vi "Server2.vi"   [LabVIEW 2013]
uses:
  <vilib>/NXT/Block Support/NXT_MessageMailbox.ctl
  <vilib>/NXT/Dual Mode Library/Display/drawText.vi
types:
  T1 = typedef "LVHSConnector.ctl" = refnum<class "BrickReference.lvclass">
  T2 = typedef "NXT_MessageMailbox.ctl" = u8
  T3 = typedef "NXT_InputPort.ctl" = u32
  T4 = typedef "MotorOutput.ctl" = u8
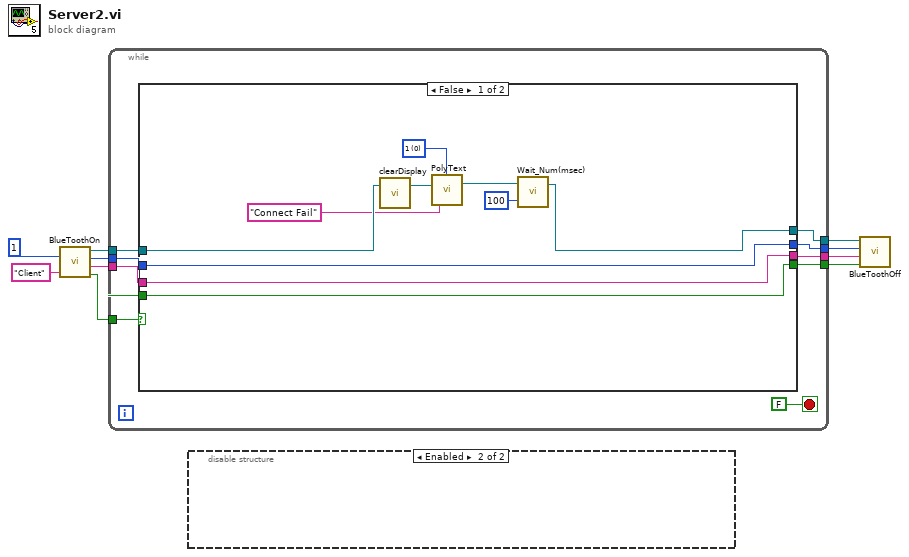
[diagram p0: block diagram]
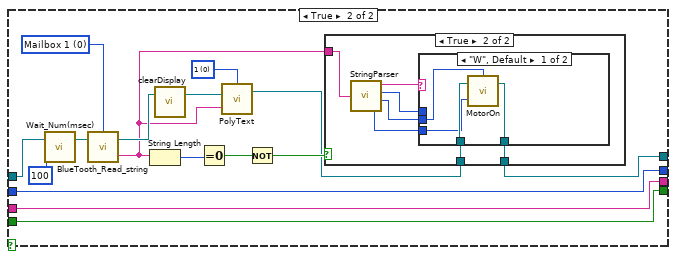
[diagram p2: hidden frame]
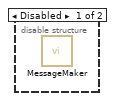
[diagram p5: hidden frame]
diagram:
  n1 = call "BlueToothOn.vi"("Connection"=u8 1, "Partner Name"="Client") -> ("NXT/EV3 2"=w2:T1, "Connection"=w4:u8, "Partner Name"=w7:string, "Success"=w9:bool)  [unwired: 1 in]
  n2 = while {
    tunnel: [w19] -> w10
    tunnel: w9 -> [w18]
    tunnel: w7 -> [w17]
    tunnel: [w16] -> w6
    tunnel: w4 -> [w15]
    tunnel: [w14] -> w3
    tunnel: w2 -> [w13]
    tunnel: [w12] -> w1
    stop <- FALSE stop-if-true
    n3 = case shown="False" w18 {
      tunnel: [w27 w45] -> w19
      tunnel: w18 -> [w27 w45]
      tunnel: w17 -> [w28 w44]
      tunnel: [w28 w44] -> w16
      tunnel: w15 -> [w29 w43]
      tunnel: [w20 w38] -> w14
      tunnel: w13 -> [w24 w37]
      tunnel: [w29 w43] -> w12
      frame False {
        w26 = i16 0 items=["1", "2", "3", "4", "5", "6", "7", "8", "9", "10", "11", "12"] ("Line")
        n4 = call <vilib>:"clearDisplay.vi"("NXT/EV3"=w24) -> ("NXT/EV3"=w25:T1)  [unwired: 3 in]
        n5 = call-poly <vilib>:"PolyText.vi"("Text"="Connect Fail", "NXT/EV3"=w25, "Line"=w26) -> ("NXT/EV3"=w21:T1)  [unwired: 1 in]
        n6 = call <vilib>:"Wait_Num(msec).vi"("Time (100 msec)"=u32 100, "NXT/EV3"=w21) -> ("NXT/EV3"=w20:T1)  [unwired: 2 in]
      }
      frame True {
        w32 = i16 0 items=["1", "2", "3", "4", "5", "6", "7", "8", "9", "10", "11", "12"] ("Line")
        w41 = T2 0 items=["Mailbox 1", "Mailbox 2", "Mailbox 3", "Mailbox 4", "Mailbox 5", "Mailbox 6", "Mailbox 7", "Mailbox 8", "Mailbox 9", "Mailbox 10"] ("Mailbox")
        n7 = call <vilib>:"Wait_Num(msec).vi"("Time (100 msec)"=u32 100, "NXT/EV3"=w37) -> ("NXT/EV3"=w36:T1)  [unwired: 2 in]
        n8 = call <vilib>:"BlueTooth_Read_string.vi"("NXT/EV3"=w36, "Mailbox"=w41) -> ("Message"=w31:string, "NXT/EV3"=w34:T1)  [unwired: 1 in]
        n9 = String Length(string=w31) -> (length=w42:i32)
        n10 = call <vilib>:"clearDisplay.vi"("NXT/EV3"=w34) -> ("NXT/EV3"=w33:T1)  [unwired: 3 in]
        n11 = Equal To 0?(x=w42) -> (x = 0?=w40:bool)
        n12 = call-poly <vilib>:"PolyText.vi"("Text"=w31, "NXT/EV3"=w33, "Line"=w32) -> ("NXT/EV3"=w30:T1)  [unwired: 1 in]
        n13 = Not(x=w40) -> (.not. x?=w39:bool)
        n14 = case shown="True" w39 {
          tunnel: w31 -> [_ w51]
          tunnel: w30 -> [w46 w53]
          tunnel: [w46 w52] -> w38
          frame False {
          }
          frame True {
            n15 = call "StringParser.vi"("Input"=w51) -> ("R/W"=w50:string, "Port (Port 1)"=w49:T3, "Output Port (All Ports)"=w48:T4, "NewValue"=w47:i32)
            n16 = case shown="\"W\", Default" w50 {
              tunnel: w53 -> [w57 w58]
              tunnel: [w56 w58] -> w52
              tunnel: w49 -> [_ _]
              tunnel: w48 -> [w55 _]
              tunnel: w47 -> [w54 _]
              frame "W", Default {
                n17 = call <vilib>:"MotorOn.vi"("Power (75)"=w54, "NXT/EV3"=w57, "Output Port (All Ports)"=w55) -> ("NXT/EV3"=w56:T1)  [unwired: 1 in]
              }
              frame "R" {
              }
            }
          }
        }
      }
    }
  }
  n18 = disable-structure shown="Enabled" {
    frame Disabled {
      n19 = call "MessageMaker.vi"() -> ()  [unwired: 4 in, 1 out]
    }
    frame Enabled {
    }
  }
  n20 = call "BlueToothOff.vi"("Connected"=w10, "Partner Name"=w6, "Connection"=w1, "NXT/EV3"=w3) -> ()  [unwired: 1 in, 3 out]
